vi "Perform Action on Target.vi"(7 "Point Ident":string, 8 "error in":errorcluster, 10 "Input":variant, 11 "ISeries Actor in":refnum<class "ISeries Actor.lvclass">) -> (0 "error out":errorcluster, 2 "Output":variant, 3 "ISeries Actor out":refnum<class "ISeries Actor.lvclass">)   [LabVIEW 2023, in "ISeries Actor.lvlib" / "ISeries Actor.lvclass"]
uses:
  ISeries Actor.lvclass
  <vilib>/Utility/error.llb/Error Cluster From Error Code.vi
  <vilib>/ErrorRing/Error Ring.xnode
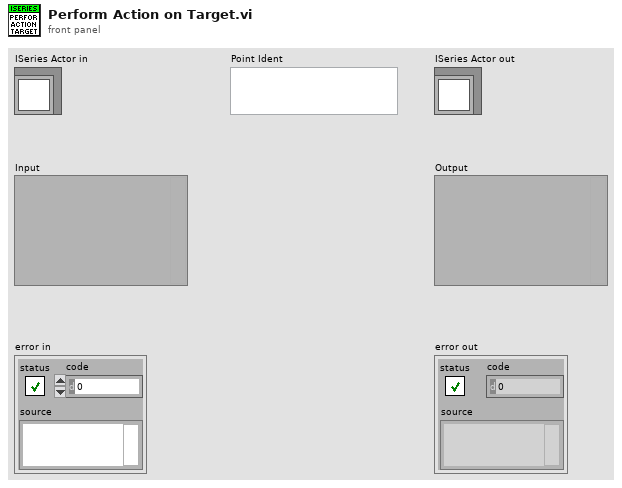
[diagram p1: front panel]
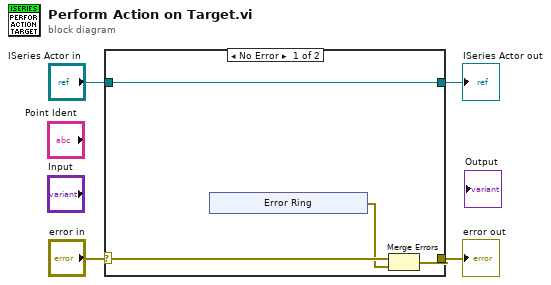
[diagram p0: block diagram]
diagram:
  n1 = case shown="No Error" "error in" {
    selector: "error in" -> [w7 w15]
    tunnel: [w6 w15] -> w3
    tunnel: [w8 w14] -> w1
    tunnel: "ISeries Actor in" -> [w8 w14]
    frame No Error {
      n2 = xnode "Error Ring"() -> ("error out"=w5:errorcluster)
      n3 = Merge Errors(w7, w5) -> (w6:errorcluster)
    }
    frame Error {
    }
  }
  "error out" <- w3
  "ISeries Actor out" <- w1
